vi "sub_apt_start.vi"(8 "错误输入（无错误）":errorcluster, 10 "HWSerialNum":i32=49871607, 11 "引用":refnum<k7>) -> (0 "错误输出":errorcluster, 3 "引用输出":refnum<k7>)   [LabVIEW 2015]
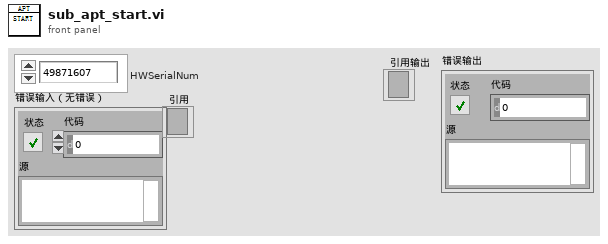
[diagram p1: front panel]
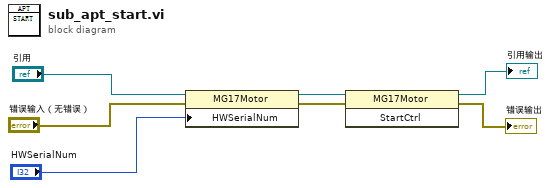
[diagram p0: block diagram]
diagram:
  n1 = property class="MG17Motor"(reference="引用", error in="错误输入（无错误）", "HWSerialNum"="HWSerialNum") -> (reference out=w7:refnum<k7>, error out=w6:errorcluster)
  n2 = invoke class="MG17Motor" method="StartCtrl"(reference=w7, error in=w6) -> (reference out=→"引用输出":refnum<k7>, error out=→"错误输出":errorcluster)  [unwired: 1 in, 1 out]
